vi "Process.vi"(8 "error in (no error)":errorcluster, 11 "Test Runner In":refnum<class "Test Runner.lvclass">) -> (0 "error out":errorcluster, 3 "Test Runner Out":refnum<class "Test Runner.lvclass">)   [LabVIEW 2020, in "Test Runner.lvclass"]
uses:
  Test Runner.lvclass
  Test Suite/LUnit Test Suite.lvclass
  Result Collector/Result Collector.lvclass
  Application Framework/Process Classes/Process/Process.lvclass
  Application Framework/Process Classes/Error Handler/Error Handler.lvclass
  Slave Test Runner/Slave Test Runner.lvclass
  C:/Git/astemes-lunit/source/Application Framework/Process Classes/Process/Process.lvclass
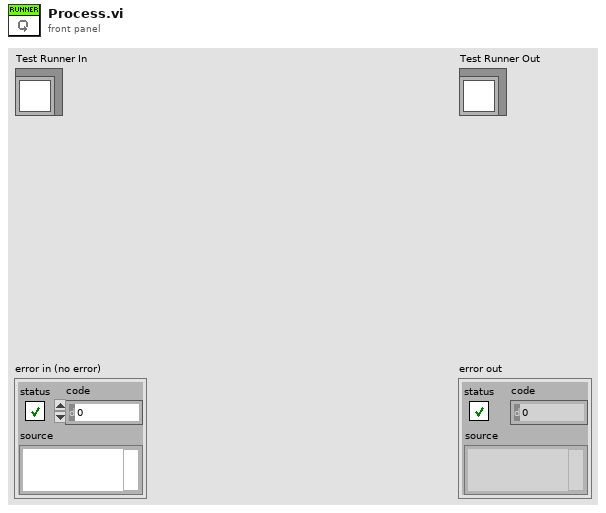
[diagram p1: front panel]
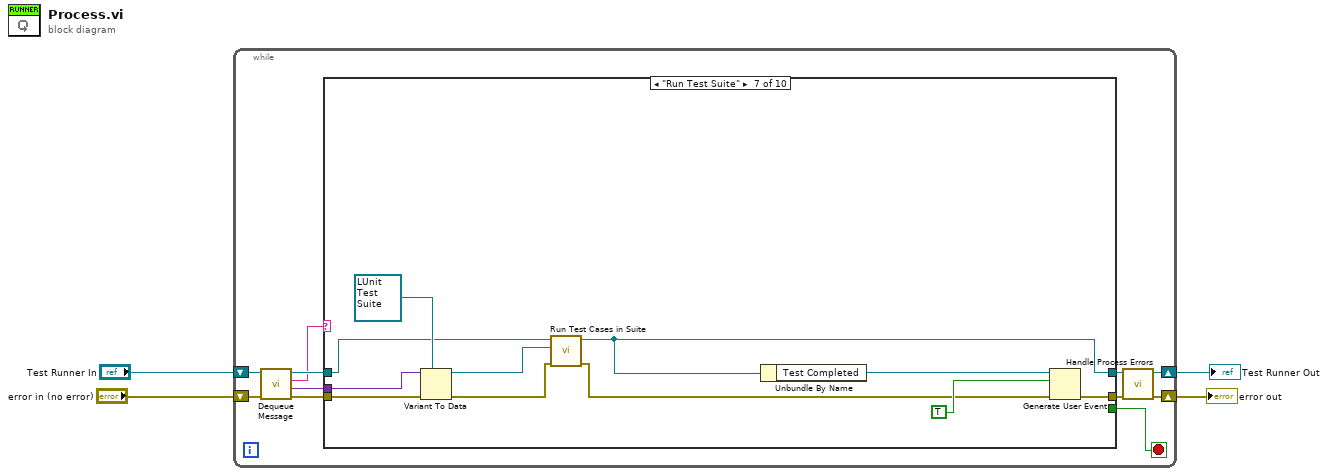
[diagram p0: block diagram]
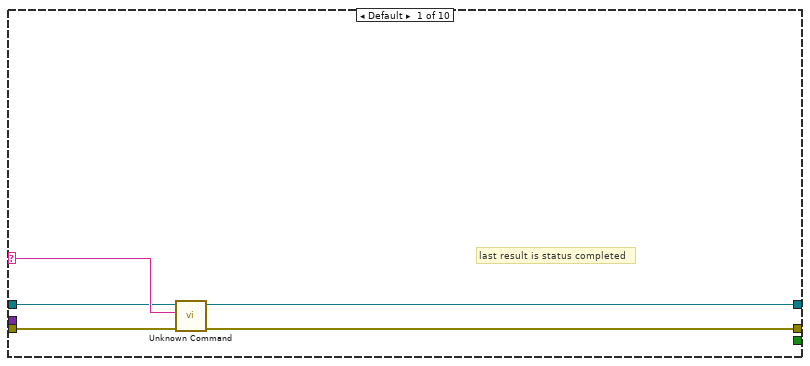
[diagram p2: hidden frame]
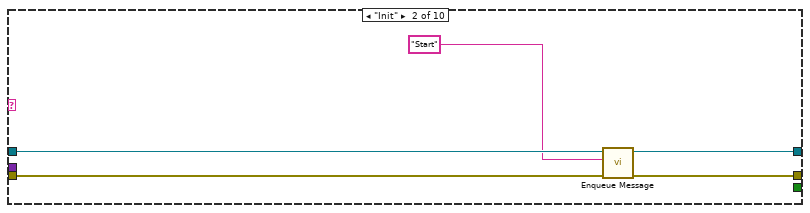
[diagram p3: hidden frame]
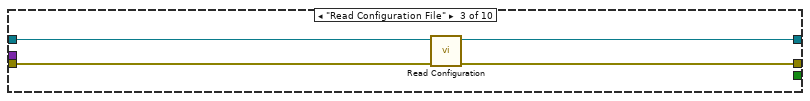
[diagram p4: hidden frame]
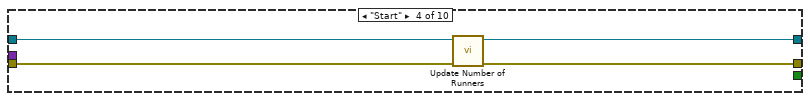
[diagram p5: hidden frame]
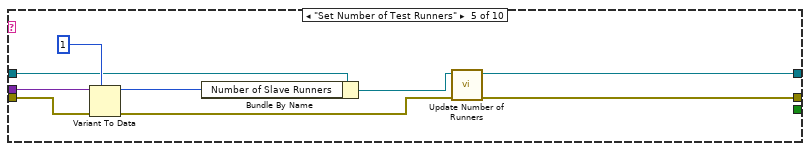
[diagram p6: hidden frame]
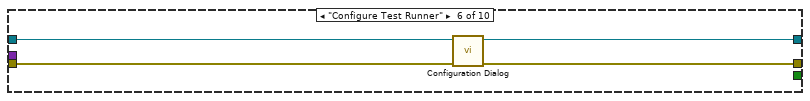
[diagram p7: hidden frame]
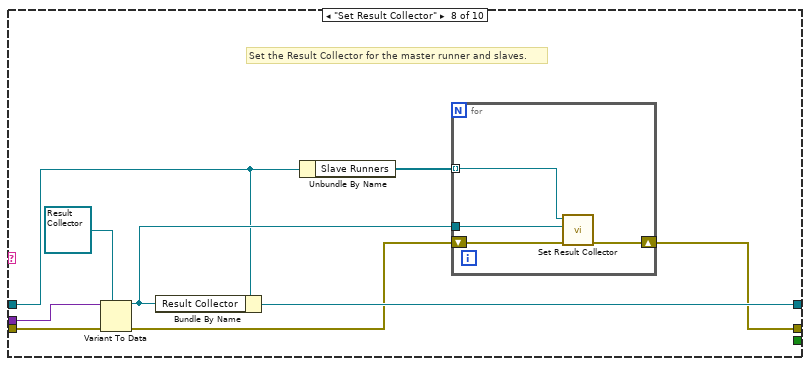
[diagram p8: hidden frame]
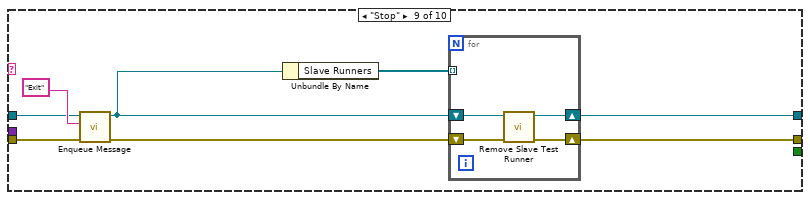
[diagram p9: hidden frame]
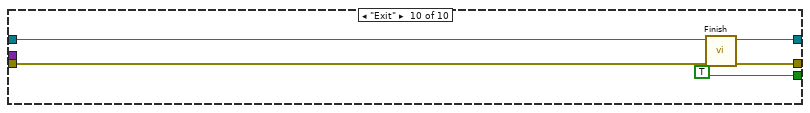
[diagram p10: hidden frame]
diagram:
  n1 = while {
    shift-right: [w5] -> w2
    shift-left: "error in (no error)" -> [w14]
    shift-right: [w7] -> w3
    shift-left: "Test Runner In" -> [w15]
    stop <- w8 stop-if-true
    n2 = call "Dequeue Message.vi"("error in (no error)"=w14, "Process In"=w15) -> ("error out"=w13:errorcluster, "Message Data"=w9:variant, "Message"=w10:string, "Process Out"=w11:refnum<class "Test Runner.lvclass">)  [unwired: 6 in]
    n3 = case shown="\"Run Test Suite\"" w10 {
      selector: w10 -> [w20 _ _ _ _ _ _ _ _ _]
      tunnel: [w17 w22 w26 w33 w36 w43 w49 w59 w75 w85] -> w6
      tunnel: w13 -> [w16 w24 w28 w32 w41 w45 w57 w66 w76 w84]
      tunnel: [w19 w23 w27 w30 w34 w44 w53 w63 w74 w86] -> w12
      tunnel: w11 -> [w18 w25 w29 w31 w39 w46 w48 w61 w77 w83]
      tunnel: w9 -> [_ _ _ _ w42 _ w56 w65 _ _]
      tunnel: [_ _ _ _ _ _ _ _ _ TRUE] -> w8
      frame Default {
        # "last result is status completed"
        n4 = call "Unknown Command.vi"("error in (no error)"=w16, "String"=w20, "Process In"=w18) -> ("error out"=w17:errorcluster, "Process Out"=w19:refnum<class "Test Runner.lvclass">)  [unwired: 7 in]
      }
      frame "Init" {
        n5 = call "Enqueue Message.vi"("error in (no error)"=w24, "Message"="Start", "Process In"=w25) -> ("error out"=w22:errorcluster, "Process Out"=w23:refnum<class "Test Runner.lvclass">)  [unwired: 7 in]
      }
      frame "Read Configuration File" {
        n6 = call-dynamic "Read Configuration.vi"("error in (no error)"=w28, "Test Runner Spawner In"=w29) -> ("error out"=w26:errorcluster, "Test Runner Spawner Out"=w27:refnum<class "Test Runner.lvclass">)  [unwired: 8 in]
      }
      frame "Start" {
        n7 = call "Update Number of Runners.vi"("error in (no error)"=w32, "Test Runner in"=w31) -> ("error out"=w33:errorcluster, "Test Runner out"=w30:refnum<class "Test Runner.lvclass">)  [unwired: 8 in]
      }
      frame "Set Number of Test Runners" {
        n8 = Variant To Data(error in=w41, type=u32 1 ("Number of Test Runners"), Variant=w42) -> (data=w38:u32, error out=w37:errorcluster)
        n9 = Bundle By Name(cluster=w39, "Number of Slave Runners"=w38) -> (w35:refnum<class "Test Runner.lvclass">)
        n10 = call "Update Number of Runners.vi"("error in (no error)"=w37, "Test Runner in"=w35) -> ("error out"=w36:errorcluster, "Test Runner out"=w34:refnum<class "Test Runner.lvclass">)  [unwired: 8 in]
      }
      frame "Configure Test Runner" {
        n11 = call "Configuration Dialog.vi"("error in (no error)"=w45, "Test Runner In"=w46) -> ("error out"=w43:errorcluster, "Test Runner Out"=w44:refnum<class "Test Runner.lvclass">)  [unwired: 8 in]
      }
      frame "Run Test Suite" {
        n12 = Variant To Data(error in=w57, type=refnum<class "LUnit Test Suite.lvclass"> refnum ("Test Suite"), Variant=w56) -> (data=w55:refnum<class "LUnit Test Suite.lvclass">, error out=w47:errorcluster)
        n13 = call "Run Test Cases in Suite.vi"("error in (no error)"=w47, "Test Suite"=w55, "Test Runner In"=w48) -> ("error out"=w50:errorcluster, "Test Runner Out"=w53:refnum<class "Test Runner.lvclass">)  [unwired: 7 in]
        n14 = Unbundle By Name(w53) -> ("Test Completed"=w52:refnum<user-event>)
        n15 = Generate User Event(user event=w52, event data cluster=TRUE ("event data"), error in=w50) -> (error out=w49:errorcluster)  [unwired: 1 in, 1 out]
      }
      frame "Set Result Collector" {
        # "Set the Result Collector for the master runner and slaves."
        n16 = Variant To Data(error in=w66, type=refnum<class "Result Collector.lvclass"> refnum ("Test Report Generator.lvclass"), Variant=w65) -> (data=w62:refnum<class "Result Collector.lvclass">, error out=w60:errorcluster)
        n17 = Bundle By Name(cluster=w61, "Result Collector"=w62) -> (w63:refnum<class "Test Runner.lvclass">)
        n18 = Unbundle By Name(w61) -> ("Slave Runners"=w58:refnum<class "Slave Test Runner.lvclass">[])
        n19 = for {
          tunnel: w62 -> [w70]
          shift-right: [w68] -> w59
          shift-left: w60 -> [w69]
          tunnel: w58 -> [w67] mode=indexing
          n20 = call "Set Result Collector.vi"("error in (no error)"=w69, "Test Suite"=w70, "Slave Test Runner In"=w67) -> ("error out"=w68:errorcluster)  [unwired: 7 in, 1 out]
        }
      }
      frame "Stop" {
        n21 = call "Enqueue Message.vi"("error in (no error)"=w76, "Message"="Exit", "Process In"=w77) -> ("error out"=w71:errorcluster, "Process Out"=w72:refnum<class "Test Runner.lvclass">)  [unwired: 7 in]
        n22 = Unbundle By Name(w72) -> ("Slave Runners"=w73:refnum<class "Slave Test Runner.lvclass">[])
        n23 = for {
          tunnel: w73 -> [_] mode=indexing
          shift-right: [w81] -> w75
          shift-left: w71 -> [w82]
          shift-right: [w80] -> w74
          shift-left: w72 -> [w79]
          n24 = call "Remove Slave Test Runner.vi"("error in (no error)"=w82, "Test Runner in"=w79) -> ("error out"=w81:errorcluster, "Test Runner out"=w80:refnum<class "Test Runner.lvclass">)  [unwired: 8 in]
        }
      }
      frame "Exit" {
        n25 = call "Finish.vi"("error in (no error)"=w84, "Process In"=w83) -> ("error out"=w85:errorcluster, "Process Out"=w86:refnum<class "Test Runner.lvclass">)  [unwired: 8 in]
      }
    }
    n26 = call "Handle Process Errors.vi"("error in (no error)"=w6, "Process In"=w12) -> ("error out"=w5:errorcluster, "Process Out"=w7:refnum<class "Test Runner.lvclass">)  [unwired: 8 in]
  }
  "error out" <- w2
  "Test Runner Out" <- w3
